vi "ReadWrite Label.vi"(5 "Mode":T13, 6 "ScheduledSDI":bool, 7 "Iteration":i32, 8 "error in (no error)":errorcluster, 10 "FIFOs In":T1, 11 "Label In":T2 {"Words"."Param Setting"."Num Bits" min=1 max=32; "Words"."Param Setting"."Start Bit" min=8 max=31; "Words"."Block Data Refs"."Data Reference" format="%.0x"; "Label" format="%.0o"}) -> (0 "error out":errorcluster, 2 "FIFOs Out":T1, 3 "Label Out":T2 {"Words"."Param Setting"."Num Bits" min=1 max=32; "Words"."Param Setting"."Start Bit" min=8 max=31; "Words"."Block Data Refs"."Data Reference" format="%.0x"; "Label" format="%.0o"})   [LabVIEW 2016, in "Ballard Arinc-429 Engine.lvlib"]
uses:
  Ballard Arinc-429 Engine.lvlib
  RT Controls/ReadWrite Selector.ctl
  RT Controls/RT Label Settings.ctl
  Shared/Controls and Global/Label.ctl
  Shared/Controls and Global/transferPeriod.ctl
  RT Controls/Driver Data.ctl
  RT Controls/RT Word Settings.ctl
  <vilib>/NI Veristand/Custom Device API/Block Data Reference.ctl
  <vilib>/NI Veristand/Custom Device API/Data Reference.ctl
  RT Controls/RT Param Setting.ctl
  Shared/Controls and Global/Start Bit.ctl
  Shared/Controls and Global/Number of Bits.ctl
  Shared/Controls and Global/TransferType.ctl
  RT Controls/FIFO.ctl
  Double to selected bits.vi
  Shared/Word to double.vi
  <vilib>/NI Veristand/Custom Device API/NI VeriStand - Get Channel Values by Block Data Reference.vi
  <vilib>/NI Veristand/Custom Device API/NI VeriStand - Set Channel Values by Block Data Reference.vi
  <vilib>/NI Veristand/Custom Device API/Global Data Refs.vi
  <instrlib>/AIT 429/Public/Tx/Data/AIT 429 Set Acyclic Transfer Data.vi
  <instrlib>/AIT 429/Public/Tx/Data/AIT 429 Get Acyclic Transfer Data.vi
  <instrlib>/AIT 429/Public/Tx/Data/AIT 429 Set Block Transfer Data.vi
  <instrlib>/AIT 429/Public/Tx/Data/AIT 429 Get Block Transfer Data.vi
  <instrlib>/AIT 429/Public/Tx/Data/AIT 429 Set Scheduled Label Data.vi
  <instrlib>/AIT 429/Public/Tx/Data/AIT 429 Get Scheduled Label Data.vi
  Shared/Ballard Arinc-429 Shared.lvlib
  <vilib>/NI Veristand/Custom Device API/Custom Device API.lvlib
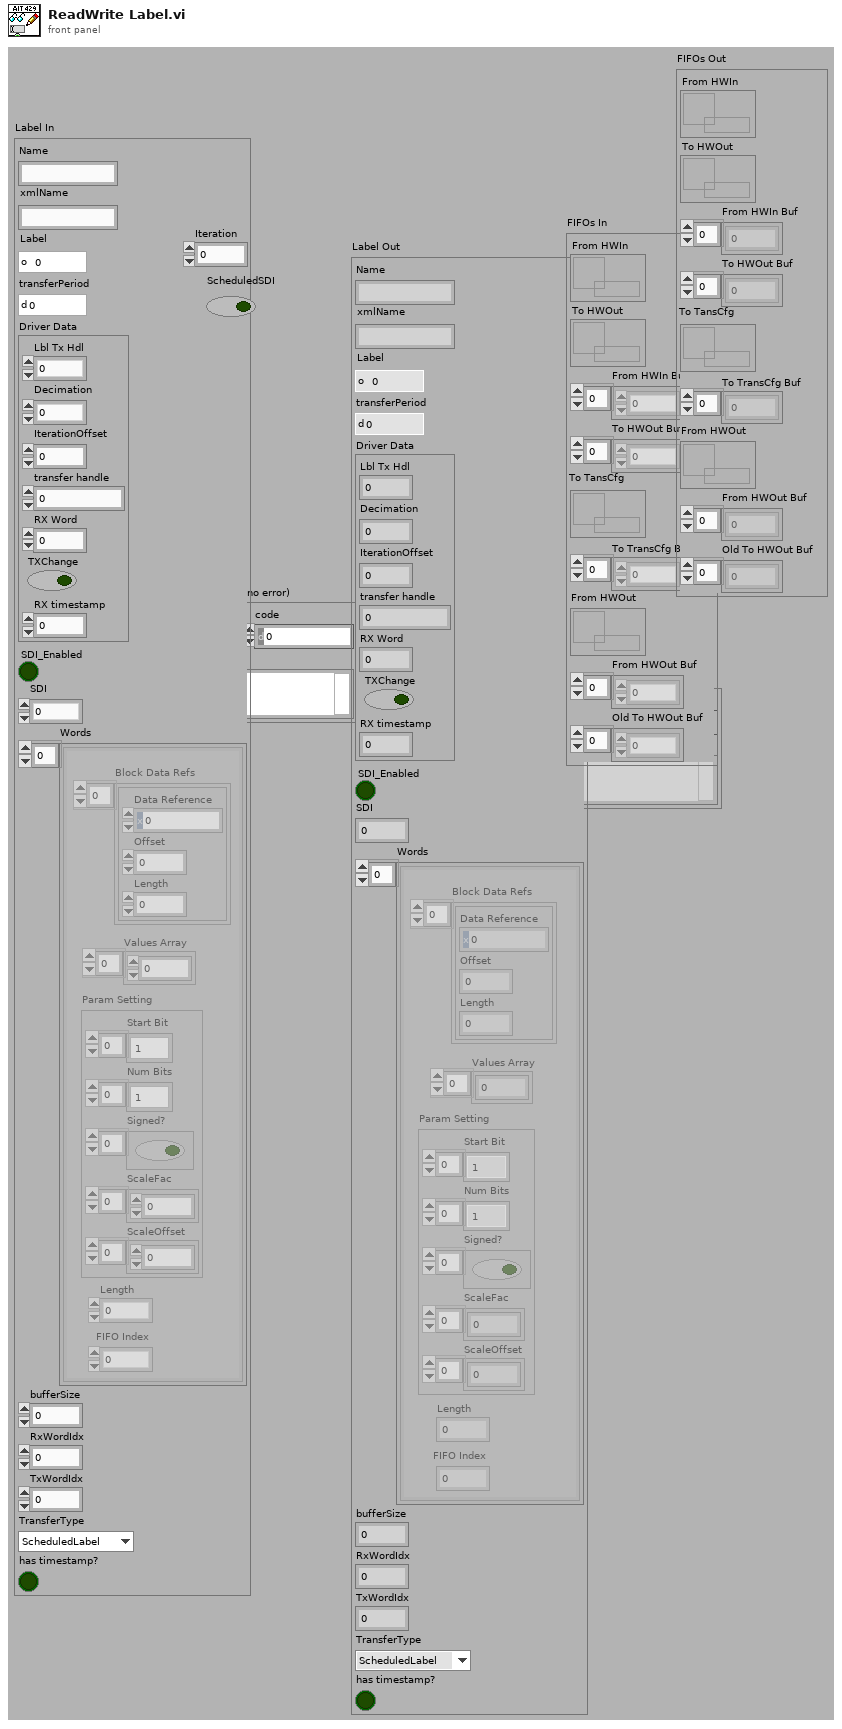
[diagram p1: front panel]
types:
  T1 = typedef "Ballard Arinc-429 Engine.lvlib/FIFO.ctl" = cluster{"From HWIn":refnum<k33>, "To HWOut":refnum<k33>, "From HWIn Buf":dbl[], "To HWOut Buf":dbl[], "To TansCfg":refnum<k33>, "To TransCfg Buf":dbl[], "From HWOut":refnum<k33>, "From HWOut Buf":dbl[], "Old To HWOut Buf":dbl[]}
  T2 = typedef "Ballard Arinc-429 Engine.lvlib/RT Label Settings.ctl" = cluster{"Name":string, "xmlName":string, "Label":T3, "transferPeriod":T4, "Driver Data":T5, "SDI_Enabled":bool, "SDI":u8, "Words":T6[], "bufferSize":u32, "RxWordIdx":i32, "TxWordIdx":i32, "TransferType":T12, "has timestamp?":bool}
  T3 = typedef "Ballard Arinc-429 Shared.lvlib/Label.ctl" = u8
  T4 = typedef "Ballard Arinc-429 Shared.lvlib/transferPeriod.ctl" = u32
  T5 = typedef "Ballard Arinc-429 Engine.lvlib/Driver Data.ctl" = cluster{"Lbl Tx Hdl":u32, "Decimation":i32, "IterationOffset":i32, "transfer handle":u32, "RX Word":u32, "TXChange":bool, "RX timestamp":dbl}
  T6 = typedef "Ballard Arinc-429 Engine.lvlib/RT Word Settings.ctl" = cluster{"Block Data Refs":T7[], "Values Array":dbl[], "Length":i32, "FIFO Index":i32, "Param Setting":T9}
  T7 = typedef "Custom Device API.lvlib/Block Data Reference.ctl" = cluster{"Data Reference":T8, "Offset":u64, "Length":u64}
  T8 = typedef "Custom Device API.lvlib/Data Reference.ctl" = i32
  T9 = typedef "Ballard Arinc-429 Engine.lvlib/RT Param Setting.ctl" = cluster{"Start Bit":T10[], "Num Bits":T11[], "Signed?":bool[], "ScaleFac":dbl[], "ScaleOffset":dbl[]}
  T10 = typedef "Ballard Arinc-429 Shared.lvlib/Start Bit.ctl" = i32
  T11 = typedef "Ballard Arinc-429 Shared.lvlib/Number of Bits.ctl" = i32
  T12 = typedef "Ballard Arinc-429 Shared.lvlib/TransferType.ctl" = enum16{"ScheduledLabel", "Acyclic", "Block", "Strobe"}
  T13 = typedef "Ballard Arinc-429 Engine.lvlib/ReadWrite Selector.ctl" = enum16{"Inline Read", "Inline Write", "Async HWIn", "Async HWOut"}
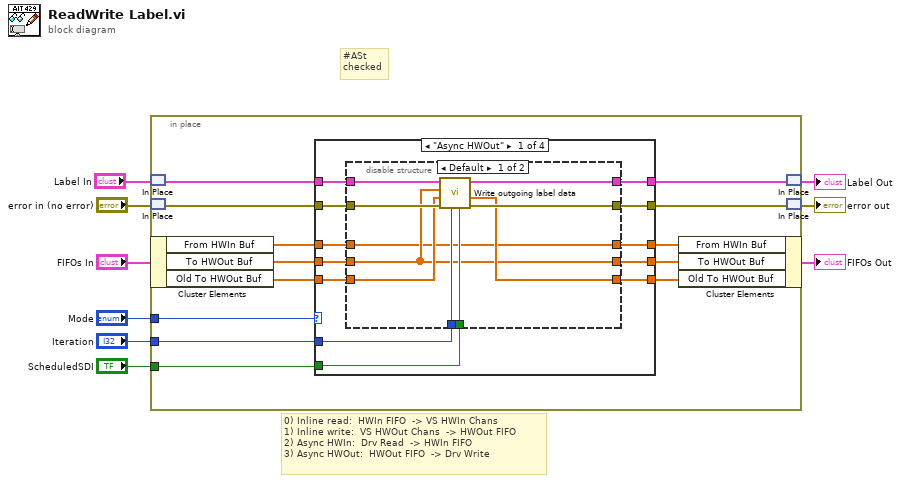
[diagram p0: block diagram]
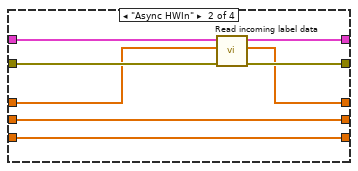
[diagram p3: hidden frame]
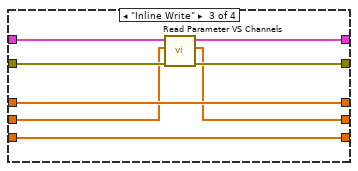
[diagram p4: hidden frame]
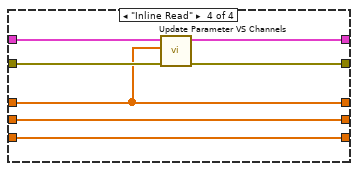
[diagram p5: hidden frame]
diagram:
  # "#ASt\nchecked"
  # "0) Inline read:\t\tHWIn FIFO \t-> VS HWIn Chans\n1) Inline write: \tVS HWOut Chans \t-> HWOut FIFO\n2) Async HWIn:\t\tDrv Read \t-> HWIn FIFO\n3) Async HWOut: \tHWOut FIFO \t-> Drv Write"
  n1 = in-place {
    in-place-border: "Mode" -> [w14]
    in-place-border: "Iteration" -> [w16]
    in-place-border: "ScheduledSDI" -> [w15]
    n2 = in-place-match #1("Label In") -> (w13:T2)
    n3 = in-place-match #2("error in (no error)") -> (w21:errorcluster)
    n4 = in-place-cluster #3("FIFOs In") -> ("From HWIn Buf"=w17:dbl[], "To HWOut Buf"=w18:dbl[], "Old To HWOut Buf"=w11:dbl[])
    n5 = case shown="\"Async HWOut\"" w14 {
      tunnel: [w34 w57 w65 w72] -> w22
      tunnel: w21 -> [w33 w56 w64 w71]
      tunnel: [w25 w55 w62 w70] -> w20
      tunnel: [w23 w51 w63 w69] -> w19
      tunnel: w18 -> [w27 w55 w59 w70]
      tunnel: w17 -> [w24 w52 w63 w69]
      tunnel: w16 -> [w32 _ _ _]
      tunnel: w15 -> [w31 _ _ _]
      tunnel: w11 -> [w28 w50 w58 w66]
      tunnel: w13 -> [w30 w54 w61 w68]
      tunnel: [w29 w53 w60 w67] -> w12
      tunnel: [w26 w50 w58 w66] -> w10
      frame "Async HWOut" {
        n6 = disable-structure shown="Default" {
          disable-tunnel: [w44 w47] -> w34
          disable-tunnel: w33 -> [w43 w47]
          disable-tunnel: w32 -> [w42 _]
          disable-tunnel: w31 -> [w41 _]
          disable-tunnel: w30 -> [w40 w48]
          disable-tunnel: [w39 w48] -> w29
          disable-tunnel: w28 -> [w38 w49]
          disable-tunnel: w27 -> [w36 w45]
          disable-tunnel: [w37 w49] -> w26
          disable-tunnel: [w36 w45] -> w25
          disable-tunnel: w24 -> [w35 w46]
          disable-tunnel: [w35 w46] -> w23
          frame condition #0 (active) {
            n7 = call "Write outgoing label data.vi"("ScheduledSDI"=w41, "Iteration"=w42, "error in (no error)"=w43, "Last iteration values"=w38, "This iteration values"=w36, "Label Settings"=w40) -> ("error out"=w44:errorcluster, "Last iteration values Out"=w37:dbl[], "Label Settings"=w39:T2)  [unwired: 3 in]
          }
          frame condition #1 {
            # "#ASt\nHW out not implemented"
          }
        }
      }
      frame "Async HWIn" {
        n8 = call "Read incoming label data.vi"("error in (no error)"=w56, "From HWIn Buf in"=w52, "Label Settings"=w54) -> ("error out"=w57:errorcluster, "From HWIn Buf out"=w51:dbl[], "Label Settings Out"=w53:T2)  [unwired: 6 in]
      }
      frame "Inline Write" {
        n9 = call "Read Parameter VS Channels.vi"("error in (no error)"=w64, "To HWOut Buf in"=w59, "Label Settings"=w61) -> ("error out"=w65:errorcluster, "To HWOut Buf out"=w62:dbl[], "Label Settings"=w60:T2)  [unwired: 6 in]
      }
      frame "Inline Read" {
        n10 = call "Update Parameter VS Channels.vi"("error in (no error)"=w71, "From HWIn Buf"=w69, "Label Settings"=w68) -> ("error out"=w72:errorcluster, "Label Settings"=w67:T2)  [unwired: 7 in]
      }
    }
    n11 = in-place-cluster #3("From HWIn Buf"=w19, "To HWOut Buf"=w20, "Old To HWOut Buf"=w10) -> (→"FIFOs Out":T1)
    n12 = in-place-match #1(w12) -> (→"Label Out":T2)
    n13 = in-place-match #2(w22) -> (→"error out":errorcluster)
  }
